vi "SW_Get_temporary_save_path.vi"(3 "Temporary file name prefix":string="TrackTemp") -> (0 "Temporary file output path":path, 1 "date/time string":string)   [LabVIEW 2016]
uses:
  <vilib>/Utility/sysdir.llb/System Directory Type.ctl
panel:
  in  "error in (no error)":errorcluster
  out "error out":errorcluster
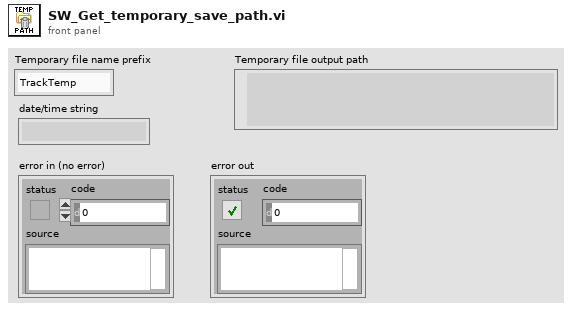
[diagram p1: front panel]
types:
  T1 = typedef "System Directory Type.ctl" = i32
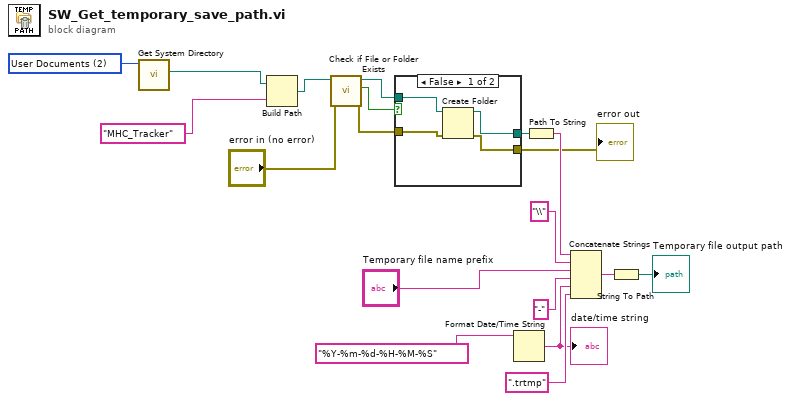
[diagram p0: block diagram]
diagram:
  w10 = T1 2 items=["User Home"=0, "User Desktop"=1, "User Documents"=2, "User Application Data"=3, "User Preferences"=4, "User Temporary"=5, "Public Documents"=6, "Public Application Data"=7, "Public Preferences"=8, "Public Cache"=13, "System Core Libraries"=9, "System Installed Libraries"=10, "Application Files"=11, "Boot Volume Root"=12] ("system directory type")
  n1 = call <vilib>:"Get System Directory.vi"("system directory type"=w10) -> ("system directory"=w8:path)  [unwired: 10 in]
  n2 = Build Path(base path=w8, name or relative path="MHC_Tracker" ("string")) -> (appended path=w7:path)
  n3 = call <vilib>:"Check if File or Folder Exists.vi"("error in (no error)"="error in (no error)", "path"=w7) -> ("error out"=w4:errorcluster, "file or folder exists?"=w6:bool, "dup path"=w5:path)  [unwired: 7 in]
  n4 = case shown="False" w6 {
    tunnel: w5 -> [w22 w25]
    tunnel: w4 -> [w23 w24]
    tunnel: [w21 w25] -> w3
    tunnel: [w20 w24] -> w2
    frame False {
      n5 = Create Folder(path (use dialog)=w22, error in=w23) -> (created path=w21:path, error out=w20:errorcluster)  [unwired: 1 in, 1 out]
    }
    frame True {
    }
  }
  "error out" <- w2
  n6 = Format Date/Time String(time format string (%c)="%Y-%m-%d-%H-%M-%S") -> (date/time string=w11:string)  [unwired: 2 in]
  "date/time string" <- w11
  n7 = Path To String(path=w3) -> (string=w17:string)
  n8 = Concatenate Strings(w17, "\\" ("string"), "Temporary file name prefix", "-" ("string"), w11, ".trtmp" ("string")) -> (w19:string)
  n9 = String To Path(string=w19) -> (path=→"Temporary file output path":path)
